vi "SetAiAlarms.vi"(0 "reference in":refnum<class "Stand.lvclass">, 11 "error in (no error)":errorcluster) -> (4 "reference out":refnum<class "Stand.lvclass">, 15 "error out":errorcluster)   [LabVIEW 2019, in "Stand.lvclass"]
uses:
  Stand.lvclass
  TypeDef/ConfigAnalogComp.ctl
  AI_class/AI.lvclass
  TypeDef/GUI Alarm developer settings.ctl
  TypeDef/GUI Alarm customer settings.ctl
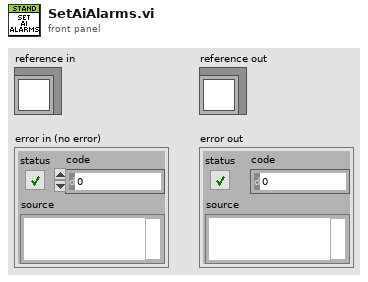
[diagram p1: front panel]
types:
  T1 = typedef "ConfigAnalogComp.ctl" = cluster{"Threshold":dbl, "Hysteresis":dbl, "Invert":bool, "Enable":bool, "LockEn":bool}
  T2 = enum16{"RAW MAX", "RAW MIN", "HIHI", "HI", "LO", "LOLO"}
  T3 = typedef "GUI Alarm customer settings.ctl" = cluster{"HIHI AI2":dbl, "HI AI2":dbl, "HIHI AI3":dbl, "HI AI3":dbl, "ENG0 OFF TIMEOUT":dbl, "ENG0 ON TIMEOUT":dbl, "HIHI AI7":dbl, "HI AI7":dbl, "HIHI AI6":dbl, "HI AI6":dbl, "HIHI AI5":dbl, "HI AI5":dbl}
  T4 = typedef "GUI Alarm developer settings.ctl" = cluster{"HIHI AI2":dbl, "HI AI2":dbl, "HIHI AI0":dbl, "HI AI0":dbl, "LOLO AI0":dbl, "LO AI0":dbl, "ENG2 OFF TIMEOUT":dbl, "ENG2 ON TIMEOUT":dbl, "HIHI AI3":dbl, "HI AI3":dbl, "HIHI AI1":dbl, "HI AI1":dbl, "LOLO AI1":dbl, "LO AI1":dbl, "ENG1 OFF TIMEOUT":dbl, "ENG1 ON TIMEOUT":dbl, "ENG0 OFF TIMEOUT":dbl, "ENG0 ON TIMEOUT":dbl, "LOLO AI8":dbl, "LO AI8":dbl, "LOLO AI9":dbl, "LO AI9":dbl, "LOLO AI5":dbl, "LO AI5":dbl, "Out Of Range HI":dbl, "Out Of Range LO":dbl}
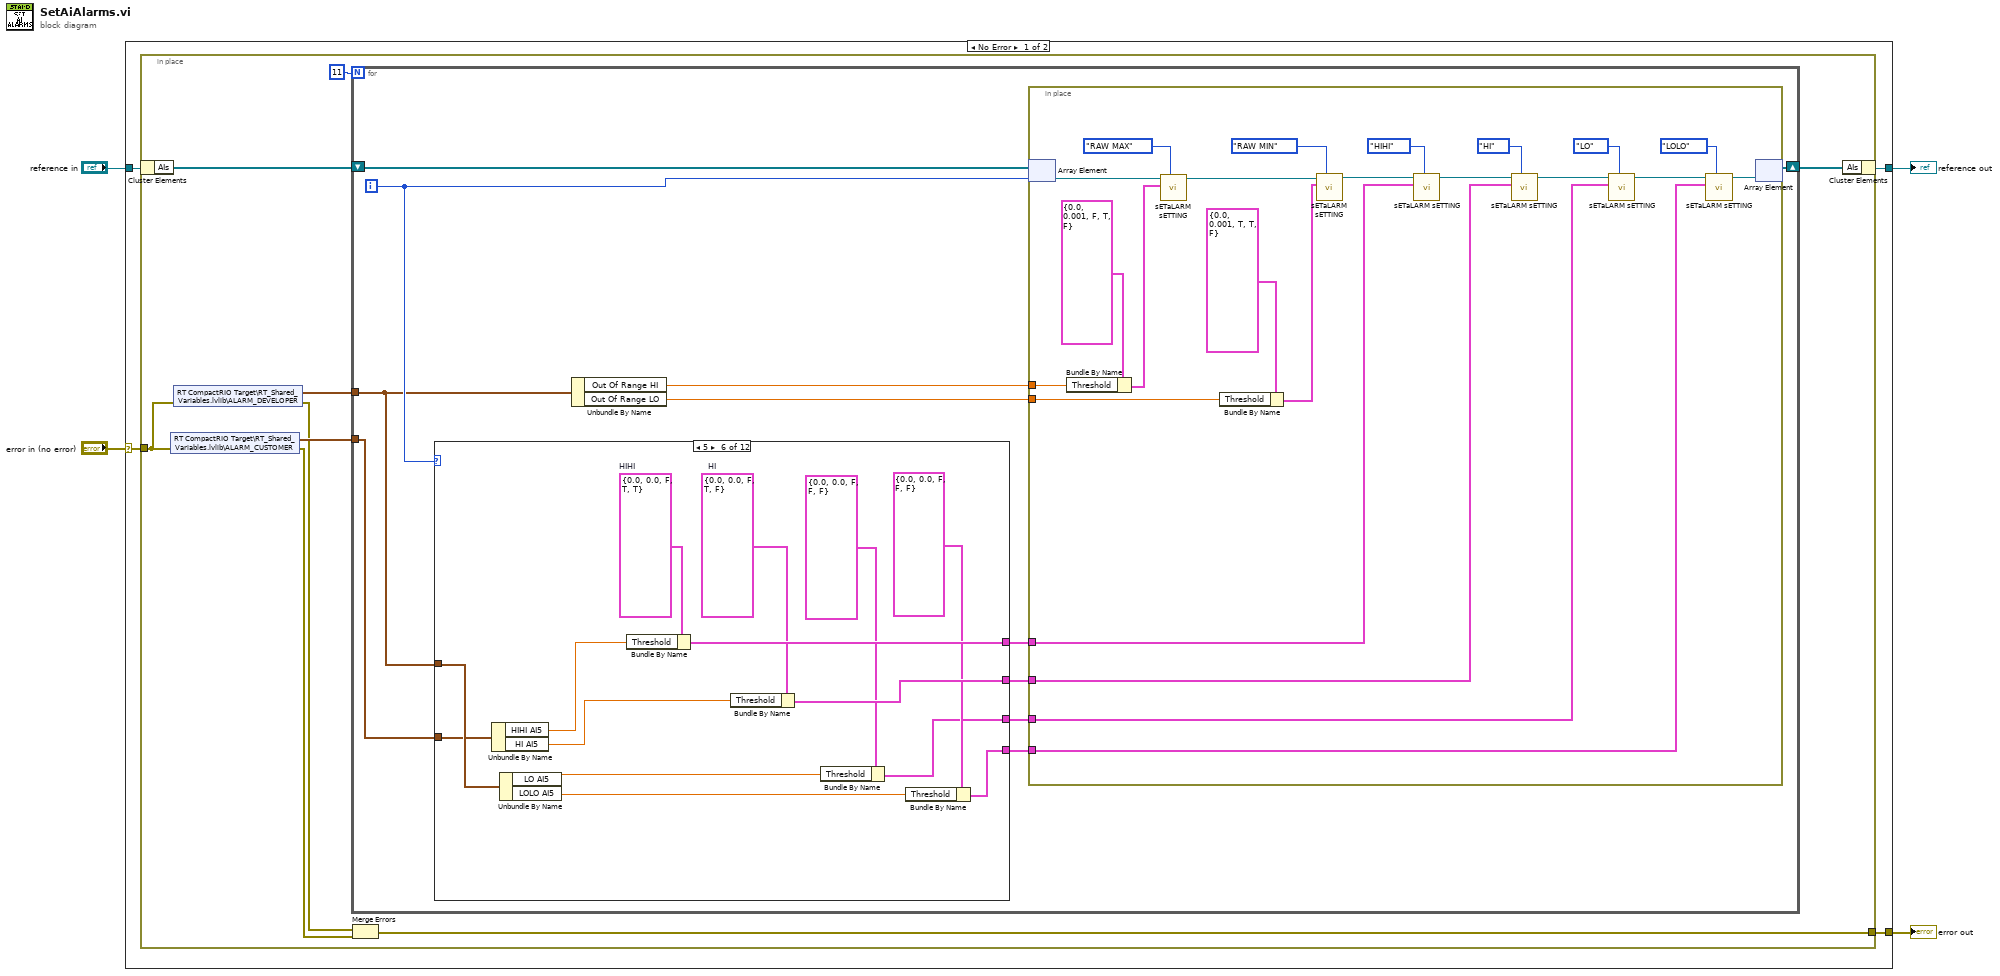
[diagram p0: block diagram]
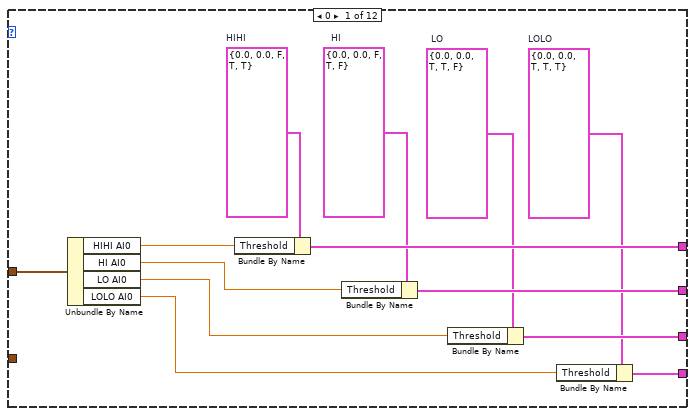
[diagram p2: hidden frame]
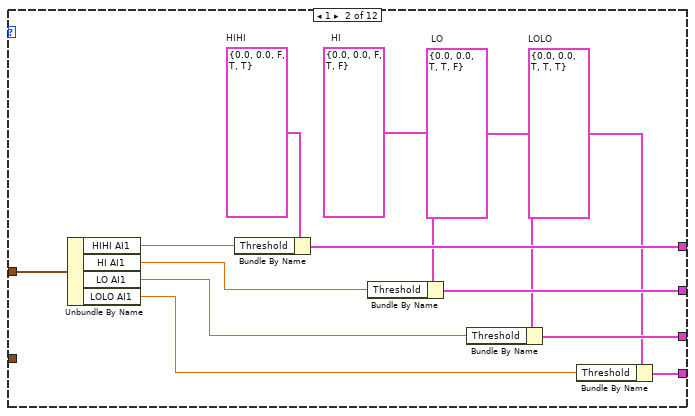
[diagram p3: hidden frame]
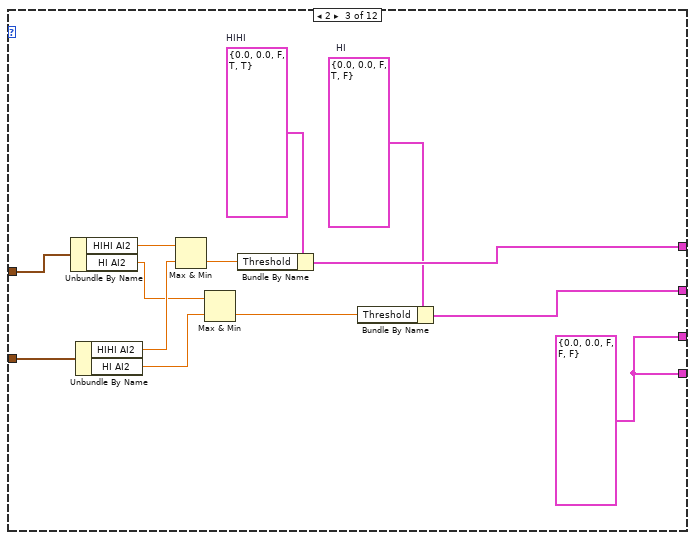
[diagram p4: hidden frame]
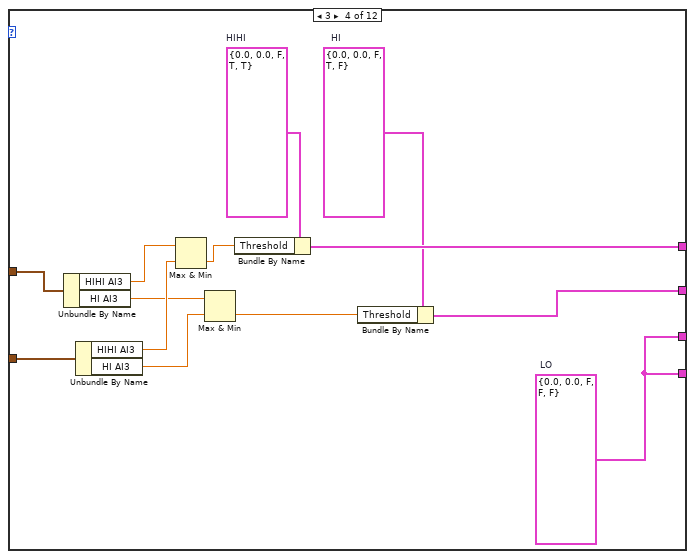
[diagram p5: hidden frame]
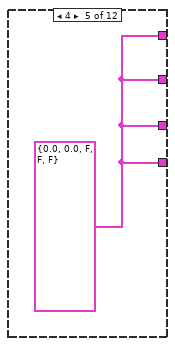
[diagram p6: hidden frame]
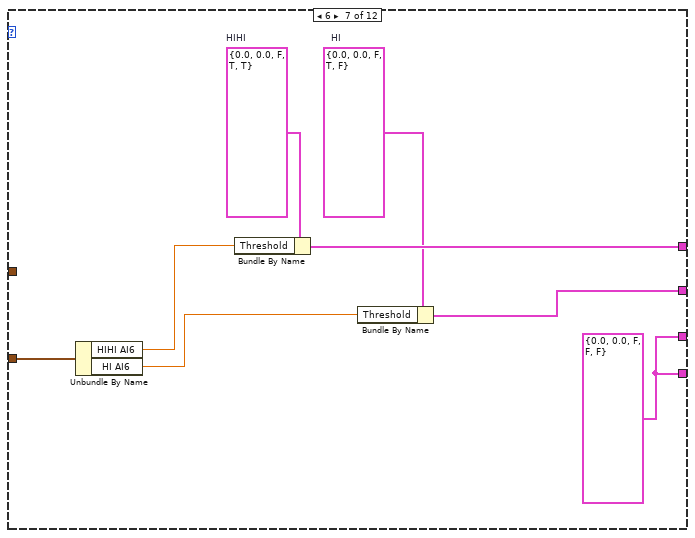
[diagram p7: hidden frame]
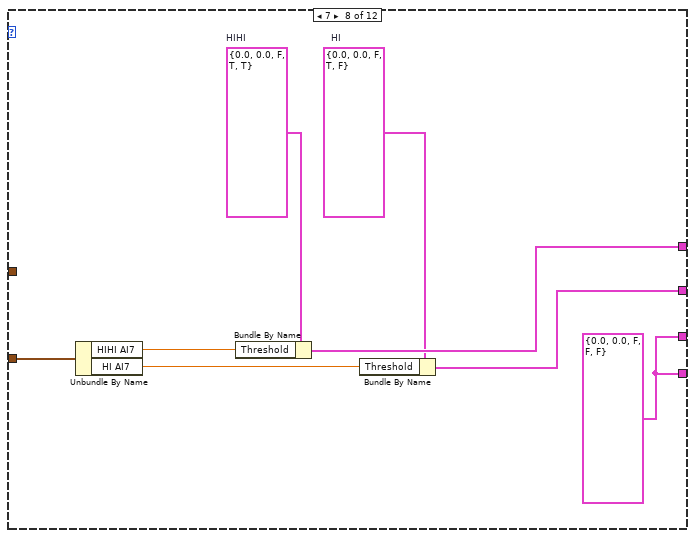
[diagram p8: hidden frame]
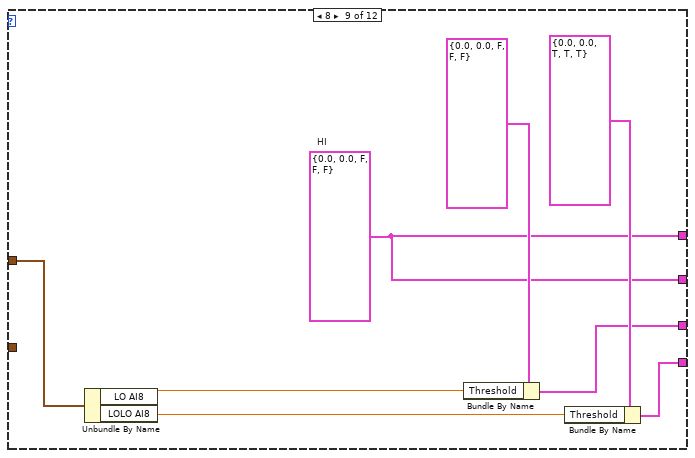
[diagram p9: hidden frame]
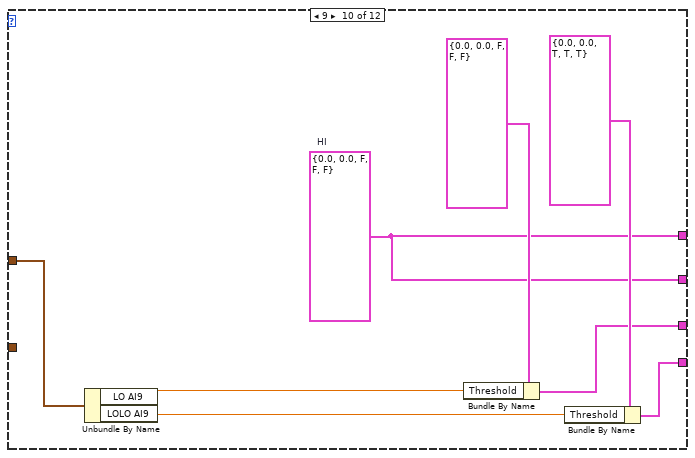
[diagram p10: hidden frame]
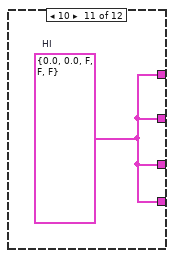
[diagram p11: hidden frame]
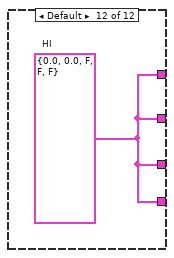
[diagram p12: hidden frame]
diagram:
  n1 = case shown="No Error" "error in (no error)" {
    selector: "error in (no error)" -> [w8 w154]
    tunnel: [w5 w154] -> w3
    tunnel: [w6 w153] -> w2
    tunnel: "reference in" -> [w7 w153]
    frame No Error {
      n2 = in-place {
        in-place-border: w8 -> [w16]
        in-place-border: [w11] -> w5
        n3 = in-place-cluster #1(w7) -> ("AIs"=w17:refnum<class "AI.lvclass">[])
        n4 = shared-variable "RT CompactRIO Target\\RT_Shared_Variables.lvlib\\ALARM_CUSTOMER"(error in=w16) -> (w14:T3, error out=w12:errorcluster)
        n5 = shared-variable "RT CompactRIO Target\\RT_Shared_Variables.lvlib\\ALARM_DEVELOPER"(error in=w16) -> (w13:T4, error out=w10:errorcluster)
        n6 = for {
          N: 11 -> [_]
          shift-right: [w27] -> w15
          shift-left: w17 -> [w28]
          tunnel: w14 -> [w18]
          tunnel: w13 -> [w19]
          i -> [w24]
          n7 = case shown="5" w24 {
            tunnel: [w40 w53 w66 w79 w81 w94 w102 w110 w112 w120 w128 w129] -> w23
            tunnel: [w38 w51 w64 w77 w81 w92 w100 w108 w112 w120 w128 w129] -> w22
            tunnel: [w36 w49 w55 w68 w81 w85 w96 w104 w116 w124 w128 w129] -> w21
            tunnel: [w34 w47 w55 w68 w81 w82 w96 w104 w113 w121 w128 w129] -> w20
            tunnel: w19 -> [w33 w46 w63 w76 _ w91 _ _ w119 w127 _ _]
            tunnel: w18 -> [_ _ w62 w75 _ w90 w99 w107 _ _ _ _]
            frame 0 {
              w35 = T1 {"Threshold"=0.0, "Hysteresis"=0.0, "Invert"=TRUE, "Enable"=TRUE, "LockEn"=TRUE}  # LOLO
              w37 = T1 {"Threshold"=0.0, "Hysteresis"=0.0, "Invert"=TRUE, "Enable"=TRUE, "LockEn"=FALSE}  # LO
              w39 = T1 {"Threshold"=0.0, "Hysteresis"=0.0, "Invert"=FALSE, "Enable"=TRUE, "LockEn"=FALSE}  # HI
              w41 = T1 {"Threshold"=0.0, "Hysteresis"=0.0, "Invert"=FALSE, "Enable"=TRUE, "LockEn"=TRUE}  # HIHI
              n8 = Unbundle By Name(w33) -> ("HIHI AI0"=w32:dbl, "HI AI0"=w31:dbl, "LO AI0"=w30:dbl, "LOLO AI0"=w29:dbl)
              n9 = Bundle By Name(cluster=w41, "Threshold"=w32) -> (w40:T1)
              n10 = Bundle By Name(cluster=w39, "Threshold"=w31) -> (w38:T1)
              n11 = Bundle By Name(cluster=w37, "Threshold"=w30) -> (w36:T1)
              n12 = Bundle By Name(cluster=w35, "Threshold"=w29) -> (w34:T1)
            }
            frame 1 {
              w48 = T1 {"Threshold"=0.0, "Hysteresis"=0.0, "Invert"=TRUE, "Enable"=TRUE, "LockEn"=TRUE}  # LOLO
              w50 = T1 {"Threshold"=0.0, "Hysteresis"=0.0, "Invert"=TRUE, "Enable"=TRUE, "LockEn"=FALSE}  # LO
              w52 = T1 {"Threshold"=0.0, "Hysteresis"=0.0, "Invert"=FALSE, "Enable"=TRUE, "LockEn"=FALSE}  # HI
              w54 = T1 {"Threshold"=0.0, "Hysteresis"=0.0, "Invert"=FALSE, "Enable"=TRUE, "LockEn"=TRUE}  # HIHI
              n13 = Unbundle By Name(w46) -> ("HIHI AI1"=w45:dbl, "HI AI1"=w44:dbl, "LO AI1"=w43:dbl, "LOLO AI1"=w42:dbl)
              n14 = Bundle By Name(cluster=w54, "Threshold"=w45) -> (w53:T1)
              n15 = Bundle By Name(cluster=w52, "Threshold"=w44) -> (w51:T1)
              n16 = Bundle By Name(cluster=w50, "Threshold"=w43) -> (w49:T1)
              n17 = Bundle By Name(cluster=w48, "Threshold"=w42) -> (w47:T1)
            }
            frame 2 {
              w55 = T1 {"Threshold"=0.0, "Hysteresis"=0.0, "Invert"=FALSE, "Enable"=FALSE, "LockEn"=FALSE}
              w65 = T1 {"Threshold"=0.0, "Hysteresis"=0.0, "Invert"=FALSE, "Enable"=TRUE, "LockEn"=FALSE}  # HI
              w67 = T1 {"Threshold"=0.0, "Hysteresis"=0.0, "Invert"=FALSE, "Enable"=TRUE, "LockEn"=TRUE}  # HIHI
              n18 = Unbundle By Name(w63) -> ("HIHI AI2"=w61:dbl, "HI AI2"=w58:dbl)
              n19 = Unbundle By Name(w62) -> ("HIHI AI2"=w60:dbl, "HI AI2"=w57:dbl)
              n20 = Max & Min(x=w61, y=w60) -> (min(x,y)=w59:dbl)  [unwired: 1 out]
              n21 = Max & Min(x=w58, y=w57) -> (min(x,y)=w56:dbl)  [unwired: 1 out]
              n22 = Bundle By Name(cluster=w67, "Threshold"=w59) -> (w66:T1)
              n23 = Bundle By Name(cluster=w65, "Threshold"=w56) -> (w64:T1)
            }
            frame 3 {
              w68 = T1 {"Threshold"=0.0, "Hysteresis"=0.0, "Invert"=FALSE, "Enable"=FALSE, "LockEn"=FALSE}  # LO
              w78 = T1 {"Threshold"=0.0, "Hysteresis"=0.0, "Invert"=FALSE, "Enable"=TRUE, "LockEn"=FALSE}  # HI
              w80 = T1 {"Threshold"=0.0, "Hysteresis"=0.0, "Invert"=FALSE, "Enable"=TRUE, "LockEn"=TRUE}  # HIHI
              n24 = Unbundle By Name(w76) -> ("HIHI AI3"=w74:dbl, "HI AI3"=w71:dbl)
              n25 = Unbundle By Name(w75) -> ("HIHI AI3"=w73:dbl, "HI AI3"=w70:dbl)
              n26 = Max & Min(x=w74, y=w73) -> (min(x,y)=w72:dbl)  [unwired: 1 out]
              n27 = Max & Min(x=w71, y=w70) -> (min(x,y)=w69:dbl)  [unwired: 1 out]
              n28 = Bundle By Name(cluster=w80, "Threshold"=w72) -> (w79:T1)
              n29 = Bundle By Name(cluster=w78, "Threshold"=w69) -> (w77:T1)
            }
            frame 4 {
              w81 = T1 {"Threshold"=0.0, "Hysteresis"=0.0, "Invert"=FALSE, "Enable"=FALSE, "LockEn"=FALSE}
            }
            frame 5 {
              w93 = T1 {"Threshold"=0.0, "Hysteresis"=0.0, "Invert"=FALSE, "Enable"=TRUE, "LockEn"=FALSE}  # HI
              w95 = T1 {"Threshold"=0.0, "Hysteresis"=0.0, "Invert"=FALSE, "Enable"=TRUE, "LockEn"=TRUE}  # HIHI
              n30 = Unbundle By Name(w90) -> ("HIHI AI5"=w89:dbl, "HI AI5"=w88:dbl)
              n31 = Unbundle By Name(w91) -> ("LO AI5"=w84:dbl, "LOLO AI5"=w83:dbl)
              n32 = Bundle By Name(cluster=w95, "Threshold"=w89) -> (w94:T1)
              n33 = Bundle By Name(cluster=w93, "Threshold"=w88) -> (w92:T1)
              n34 = Bundle By Name(cluster=T1 {"Threshold"=0.0, "Hysteresis"=0.0, "Invert"=FALSE, "Enable"=FALSE, "LockEn"=FALSE}, "Threshold"=w84) -> (w85:T1)
              n35 = Bundle By Name(cluster=T1 {"Threshold"=0.0, "Hysteresis"=0.0, "Invert"=FALSE, "Enable"=FALSE, "LockEn"=FALSE}, "Threshold"=w83) -> (w82:T1)
            }
            frame 6 {
              w96 = T1 {"Threshold"=0.0, "Hysteresis"=0.0, "Invert"=FALSE, "Enable"=FALSE, "LockEn"=FALSE}
              w101 = T1 {"Threshold"=0.0, "Hysteresis"=0.0, "Invert"=FALSE, "Enable"=TRUE, "LockEn"=FALSE}  # HI
              w103 = T1 {"Threshold"=0.0, "Hysteresis"=0.0, "Invert"=FALSE, "Enable"=TRUE, "LockEn"=TRUE}  # HIHI
              n36 = Unbundle By Name(w99) -> ("HIHI AI6"=w98:dbl, "HI AI6"=w97:dbl)
              n37 = Bundle By Name(cluster=w103, "Threshold"=w98) -> (w102:T1)
              n38 = Bundle By Name(cluster=w101, "Threshold"=w97) -> (w100:T1)
            }
            frame 7 {
              w104 = T1 {"Threshold"=0.0, "Hysteresis"=0.0, "Invert"=FALSE, "Enable"=FALSE, "LockEn"=FALSE}
              w109 = T1 {"Threshold"=0.0, "Hysteresis"=0.0, "Invert"=FALSE, "Enable"=TRUE, "LockEn"=FALSE}  # HI
              w111 = T1 {"Threshold"=0.0, "Hysteresis"=0.0, "Invert"=FALSE, "Enable"=TRUE, "LockEn"=TRUE}  # HIHI
              n39 = Unbundle By Name(w107) -> ("HIHI AI7"=w106:dbl, "HI AI7"=w105:dbl)
              n40 = Bundle By Name(cluster=w111, "Threshold"=w106) -> (w110:T1)
              n41 = Bundle By Name(cluster=w109, "Threshold"=w105) -> (w108:T1)
            }
            frame 8 {
              w112 = T1 {"Threshold"=0.0, "Hysteresis"=0.0, "Invert"=FALSE, "Enable"=FALSE, "LockEn"=FALSE}  # HI
              n42 = Unbundle By Name(w119) -> ("LO AI8"=w115:dbl, "LOLO AI8"=w114:dbl)
              n43 = Bundle By Name(cluster=T1 {"Threshold"=0.0, "Hysteresis"=0.0, "Invert"=FALSE, "Enable"=FALSE, "LockEn"=FALSE}, "Threshold"=w115) -> (w116:T1)
              n44 = Bundle By Name(cluster=T1 {"Threshold"=0.0, "Hysteresis"=0.0, "Invert"=TRUE, "Enable"=TRUE, "LockEn"=TRUE}, "Threshold"=w114) -> (w113:T1)
            }
            frame 9 {
              w120 = T1 {"Threshold"=0.0, "Hysteresis"=0.0, "Invert"=FALSE, "Enable"=FALSE, "LockEn"=FALSE}  # HI
              n45 = Unbundle By Name(w127) -> ("LO AI9"=w123:dbl, "LOLO AI9"=w122:dbl)
              n46 = Bundle By Name(cluster=T1 {"Threshold"=0.0, "Hysteresis"=0.0, "Invert"=FALSE, "Enable"=FALSE, "LockEn"=FALSE}, "Threshold"=w123) -> (w124:T1)
              n47 = Bundle By Name(cluster=T1 {"Threshold"=0.0, "Hysteresis"=0.0, "Invert"=TRUE, "Enable"=TRUE, "LockEn"=TRUE}, "Threshold"=w122) -> (w121:T1)
            }
            frame 10 {
              w128 = T1 {"Threshold"=0.0, "Hysteresis"=0.0, "Invert"=FALSE, "Enable"=FALSE, "LockEn"=FALSE}  # HI
            }
            frame Default {
              w129 = T1 {"Threshold"=0.0, "Hysteresis"=0.0, "Invert"=FALSE, "Enable"=FALSE, "LockEn"=FALSE}  # HI
            }
          }
          n48 = Unbundle By Name(w19) -> ("Out Of Range HI"=w26:dbl, "Out Of Range LO"=w25:dbl)
          n49 = in-place {
            in-place-border: w26 -> [w137]
            in-place-border: w25 -> [w134]
            in-place-border: w23 -> [w133]
            in-place-border: w22 -> [w132]
            in-place-border: w21 -> [w131]
            in-place-border: w20 -> [w130]
            n50 = in-place-array #2(w28, w24) -> (w152:refnum<class "AI.lvclass">)
            n51 = Bundle By Name(cluster=T1 {"Threshold"=0.0, "Hysteresis"=0.001, "Invert"=FALSE, "Enable"=TRUE, "LockEn"=FALSE} ("SettinganalogComp"), "Threshold"=w137) -> (w139:T1)
            n52 = call "sETaLARM sETTING.vi"("TYPE"=T2."RAW MAX", "SettinganalogComp"=w139, "Sig_AI in"=w152) -> ("Sig_AI out"=w150:refnum<class "AI.lvclass">)  [unwired: 8 in]
            n53 = Bundle By Name(cluster=T1 {"Threshold"=0.0, "Hysteresis"=0.001, "Invert"=TRUE, "Enable"=TRUE, "LockEn"=FALSE} ("SettinganalogComp"), "Threshold"=w134) -> (w135:T1)
            n54 = call "sETaLARM sETTING.vi"("TYPE"=T2."RAW MIN", "SettinganalogComp"=w135, "Sig_AI in"=w150) -> ("Sig_AI out"=w144:refnum<class "AI.lvclass">)  [unwired: 8 in]
            n55 = call "sETaLARM sETTING.vi"("TYPE"=T2."HIHI", "SettinganalogComp"=w133, "Sig_AI in"=w144) -> ("Sig_AI out"=w143:refnum<class "AI.lvclass">)  [unwired: 8 in]
            n56 = call "sETaLARM sETTING.vi"("TYPE"=T2."HI", "SettinganalogComp"=w132, "Sig_AI in"=w143) -> ("Sig_AI out"=w142:refnum<class "AI.lvclass">)  [unwired: 8 in]
            n57 = call "sETaLARM sETTING.vi"("TYPE"=T2."LO", "SettinganalogComp"=w131, "Sig_AI in"=w142) -> ("Sig_AI out"=w141:refnum<class "AI.lvclass">)  [unwired: 8 in]
            n58 = call "sETaLARM sETTING.vi"("TYPE"=T2."LOLO", "SettinganalogComp"=w130, "Sig_AI in"=w141) -> ("Sig_AI out"=w140:refnum<class "AI.lvclass">)  [unwired: 8 in]
            n59 = in-place-array #2(w140) -> (w27:refnum<class "AI.lvclass">[])  [unwired: 1 out]
          }
        }
        n60 = Merge Errors(w10, w12) -> (w11:errorcluster)
        n61 = in-place-cluster #1("AIs"=w15) -> (w6:refnum<class "Stand.lvclass">)
      }
    }
    frame Error {
    }
  }
  "error out" <- w3
  "reference out" <- w2
